vi "Write Entire File.vi"(5 "convert eoln (F)":bool, 8 "error in":errorcluster, 10 "data":string, 11 "path":path) -> (0 "error out":errorcluster, 3 "duplicate path":path)   [LabVIEW 2009, in "Tools_String.lvlib"]
uses:
  Tools_String.lvlib
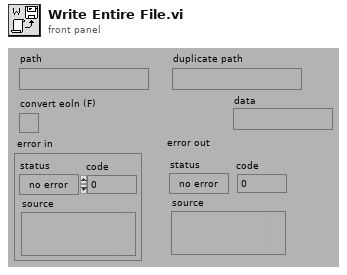
[diagram p1: front panel]
types:
  T1 = enum16{"open", "replace", "create", "open or create", "replace or create", "replace or create with confirmation"}
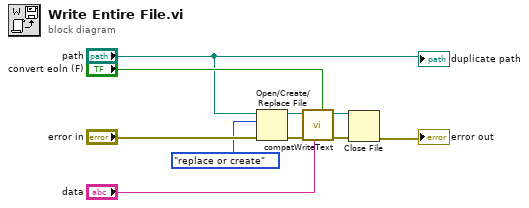
[diagram p0: block diagram]
diagram:
  n1 = Open/Create/Replace File(file path (use dialog)="path", error in="error in", operation (0:open)=T1."replace or create") -> (refnum out=w5:refnum<file>, error out=w4:errorcluster)  [unwired: 4 out]
  n2 = call <vilib>:"compatWriteText.vi"("convert eol (F)"="convert eoln (F)", "data"="data", "error in"=w4, "refnum"=w5) -> ("error out"=w9:errorcluster, "dup refnum"=w10:refnum<file>)  [unwired: 1 in, 5 out]
  n3 = Close File(refnum=w10, error in=w9) -> (error out=→"error out":errorcluster)  [unwired: 1 out]
  "duplicate path" <- "path"
